vi "Get Port Database.vi"(8 "error in":errorcluster, 11 "Port Ref":T1 format="%.0x") -> (0 "error out":errorcluster, 1 "Database Path":path, 2 "Database Name":string, 3 "Port Ref out":T1 format="%.0x", 4 "Found?":bool)   [LabVIEW 2020, in "Communication Bus Template Scripting.lvlib"]
uses:
  <vilib>/NI VeriStand/Custom Device API/Custom Device Item Ref.ctl
  Shared/Constants.vi
  Communication Bus Template Scripting.lvlib
  Shared/Communication Bus Template Shared.lvlib
  <vilib>/NI VeriStand/Custom Device API/Custom Device API.lvlib
  <vilib>/NI VeriStand/Custom Device API/Get Item Property (String).vi
  <vilib>/NI VeriStand/Custom Device API/Get Item Property (Path).vi
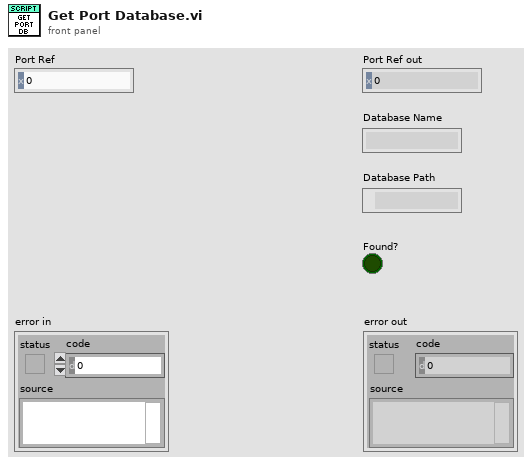
[diagram p1: front panel]
types:
  T1 = typedef "Custom Device API.lvlib/Custom Device Item Ref.ctl" = u64
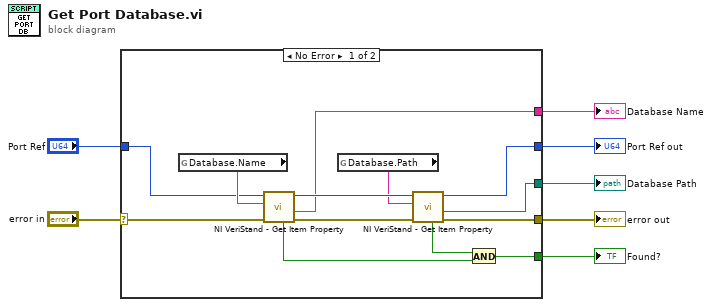
[diagram p0: block diagram]
diagram:
  n1 = case shown="No Error" "error in" {
    selector: "error in" -> [w13 w22]
    tunnel: "Port Ref" -> [w14 w21]
    tunnel: [w20 w22] -> w6
    tunnel: [w19 w21] -> w5
    tunnel: [w12 _] -> w3
    tunnel: [w11 _] -> w2
    tunnel: [w9 _] -> w1
    frame No Error {
      n2 = global read "Constants.vi" "Database.Name"() -> (w15:string)
      n3 = call-poly <vilib>:"NI VeriStand - Get Item Property.vi"("error in (no error)"=w13, "Property Name"=w15, "Item Ref in"=w14) -> ("error out"=w17:errorcluster, "Value"=w12:string, "Item Ref out"=w18:T1, "Found?"=w8:bool)  [unwired: 5 in]
      n4 = global read "Constants.vi" "Database.Path"() -> (w16:string)
      n5 = call-poly <vilib>:"NI VeriStand - Get Item Property.vi"("error in (no error)"=w17, "Property Name"=w16, "Item Ref in"=w18) -> ("error out"=w20:errorcluster, "Value"=w11:path, "Item Ref out"=w19:T1, "Found?"=w10:bool)  [unwired: 5 in]
      n6 = And(x=w10, y=w8) -> (x .and. y?=w9:bool)
    }
    frame Error {
    }
  }
  "error out" <- w6
  "Database Name" <- w3
  "Database Path" <- w2
  "Port Ref out" <- w5
  "Found?" <- w1
